vi "Initialize Sim youBot Arm.vi"(8 "error in":errorcluster, 11 "Robot ID":string) -> (0 "error out":errorcluster, 3 "NI_Robotics_KUKA youBot Arm_Sim out":refnum<class "NI_Robotics_KUKA youBot Arm_Sim.lvclass">)   [LabVIEW 2017, in "NI_Robotics_KUKA youBot Host.lvlib" / "NI_Robotics_KUKA youBot Arm_Sim.lvclass"]
uses:
  <vilib>/robotics/KUKA youBot/Basic Device/Arm Sim/NI_Robotics_KUKA youBot Arm_Sim.lvclass
  c:/Program Files (x86)/National Instruments/LabVIEW 2017/vi.lib/robotics/Kinematics/Robot/NI_Robotics_Serial Robot Arm.lvclass
  c:/Program Files (x86)/National Instruments/LabVIEW 2017/vi.lib/robotics/KUKA youBot/Basic Device/Arm/NI_Robotics_KUKA youBot Arm.lvclass
  <vilib>/robotics/Kinematics/DH Dynamic Parameters.ctl
  <vilib>/Analysis/Matrix/Datatypes/RealMatrix.ctl
  <vilib>/robotics/KUKA youBot/Motor/Arm Motor Sim/NI_Robotics_KUKA youBot Arm Motor_Sim.lvclass
  c:/Program Files (x86)/National Instruments/LabVIEW 2017/vi.lib/robotics/KUKA youBot/Motor/Arm Motor/NI_Robotics_KUKA youBot Arm Motor.lvclass
  <vilib>/robotics/KUKA youBot/Basic Device/Gripper Sim/NI_Robotics_KUKA youBot Gripper_Sim.lvclass
  c:/Program Files (x86)/National Instruments/LabVIEW 2017/vi.lib/robotics/KUKA youBot/Basic Device/Gripper/NI_Robotics_KUKA youBot Gripper.lvclass
  <vilib>/Analysis/7linalg.llb/Create Special Real Matrix.vi
  <vilib>/robotics/KUKA youBot/Basic Device/Arm/NI_Robotics_KUKA youBot Arm.lvclass
  <vilib>/robotics/Kinematics/Robot/NI_Robotics_Serial Robot Arm.lvclass
  <vilib>/robotics/Kinematics/NI_Kinematics.lvlib
  <vilib>/Analysis/NI_AALPro.lvlib
  <vilib>/Analysis/Matrix/NI_Matrix.lvlib
  <vilib>/robotics/Kinematics/Link/NI_Robotics_Link.lvclass
panel:
  in  "Arm Index":i32
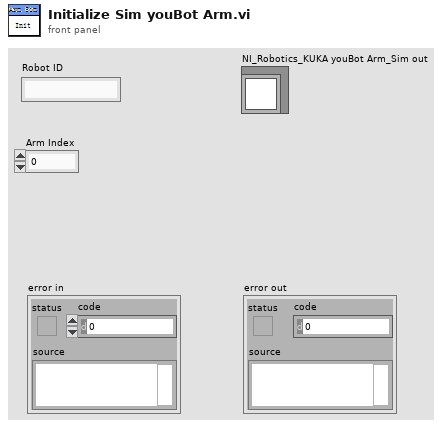
[diagram p1: front panel]
types:
  T1 = typedef "DH Dynamic Parameters.ctl" = cluster{"mass":dbl, "gear ratio":dbl, "motor inertia":dbl, "center of gravity":dbl[], "viscous friction":dbl, "positive coulomb friction":dbl, "negative coulomb friction":dbl, "inertia matrix":T2}
  T2 = typedef "NI_Matrix.lvlib/RealMatrix.ctl" = dbl[][]
  T3 = cluster{"Robot ID":string, "sensor/actuator ID":string}
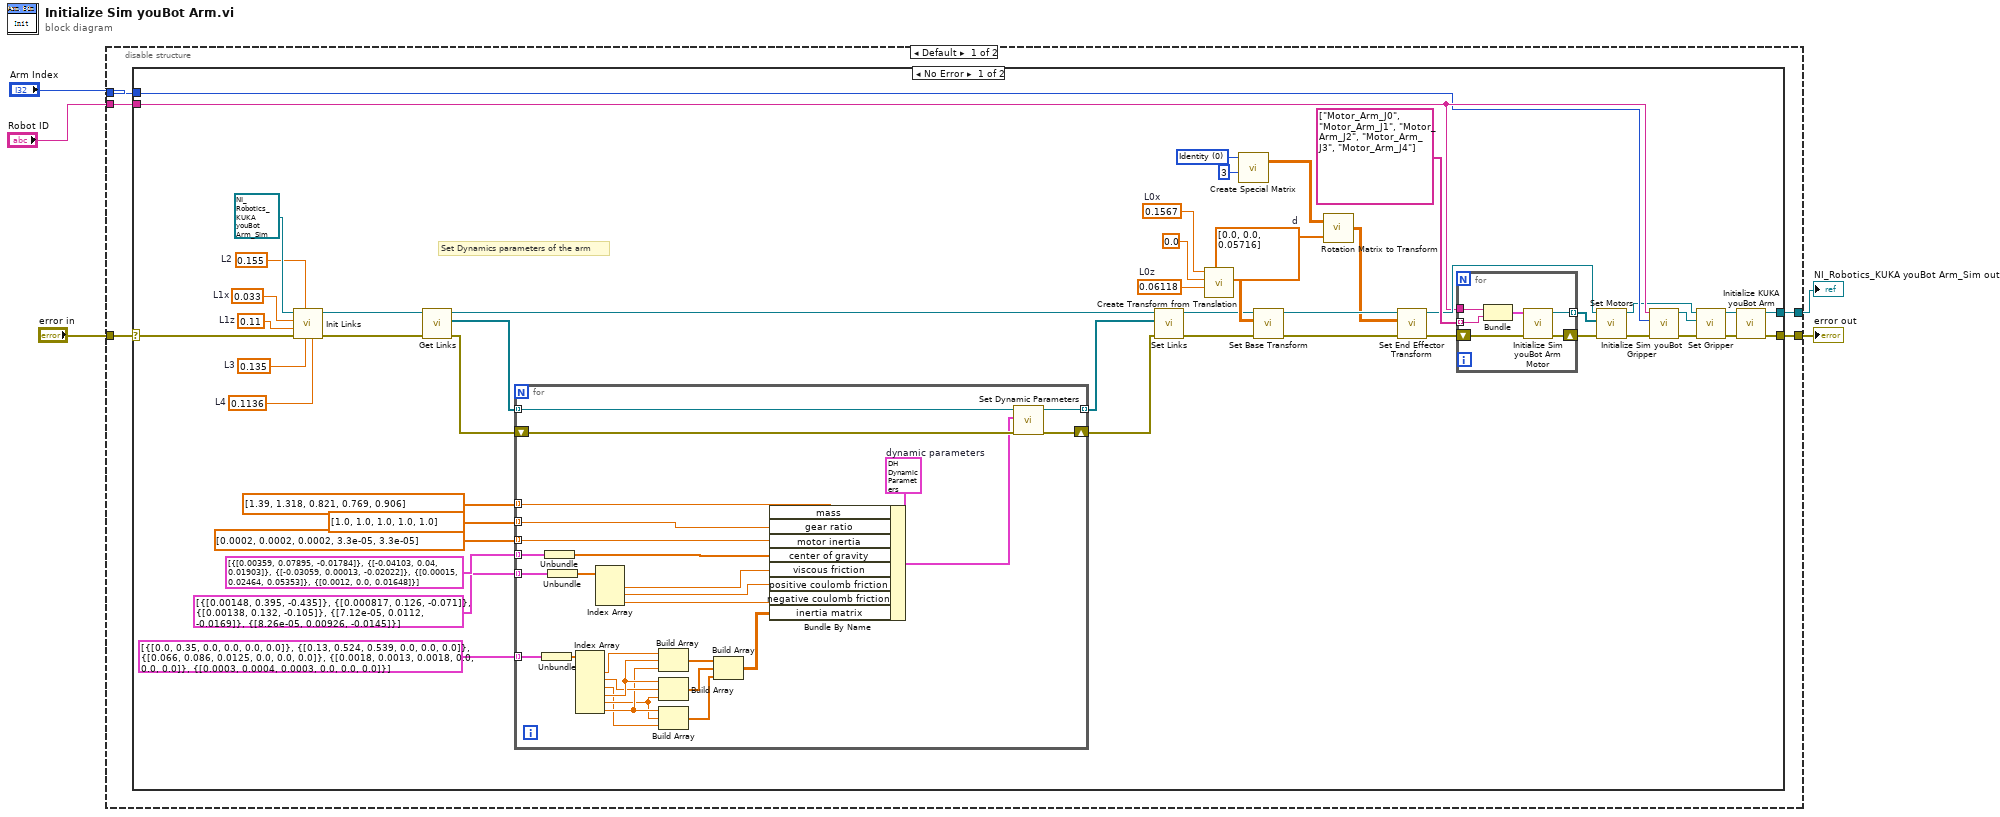
[diagram p0: block diagram]
diagram:
  n1 = disable-structure shown="Default" {
    disable-tunnel: "Robot ID" -> [w10 _]
    disable-tunnel: "error in" -> [w9 _]
    disable-tunnel: [w8 _] -> w3
    disable-tunnel: [w7 _] -> w2
    disable-tunnel: "Arm Index" -> [w6 _]
    frame condition #0 (active) {
      n2 = case shown="No Error" w9 {
        selector: w9 -> [w34 w93]
        tunnel: w10 -> [w42 _]
        tunnel: [w56 w93] -> w8
        tunnel: [w57 _] -> w7
        tunnel: w6 -> [w41 _]
        frame No Error {
          w26 = 0.1136  # L4
          w29 = 0 items=["Identity", "Diagonal", "Toeplitz", "Vandermonde", "Companion", "Hankel", "Hadamard", "Wilkinson", "Hilbert", "Inverse Hilbert", "Rosser", "Pascal"] ("matrix type")
          w44 = dbl[] [0.0, 0.0, 0.05716]  # d
          w30 = 0.135  # L3
          w31 = 0.155  # L2
          w32 = 0.11  # L1z
          w33 = 0.033  # L1x
          w50 = 0.06118  # L0z
          w52 = 0.1567  # L0x
          # "Set Dynamics parameters of the arm"
          n3 = call-dynamic "Init Links.vi"("L4"=w26, "L3"=w30, "L2"=w31, "error in (no error)"=w34, "L1z"=w32, "L1x"=w33, "NI_Robotics_5R Type 1 Serial Arm Class in"=refnum<class "NI_Robotics_KUKA youBot Arm_Sim.lvclass"> refnum ("NI_Robotics_KUKA youBot Host.lvlib:NI_Robotics_KUKA youBot Arm_Sim.lvclass")) -> ("error out"=w18:errorcluster, "NI_Robotics_5R Type 1 Serial Arm Class out"=w19:refnum<class "NI_Robotics_KUKA youBot Arm_Sim.lvclass">)  [unwired: 3 in]
          n4 = call <vilib>:"Get Links.vi"("error in (no error)"=w18, "serial arm in"=w19) -> ("error out"=w17:errorcluster, "links"=w16:refnum<class "NI_Robotics_Link.lvclass">[], "serial arm out"=w11:refnum<class "NI_Robotics_KUKA youBot Arm_Sim.lvclass">)  [unwired: 7 in]
          n5 = for {
            tunnel: w16 -> [w63] mode=indexing
            tunnel: dbl[] [1.39, 1.318, 0.821, 0.769, 0.906] -> [w85] mode=indexing
            tunnel: dbl[] [1.0, 1.0, 1.0, 1.0, 1.0] -> [w84] mode=indexing
            tunnel: dbl[] [0.0002, 0.0002, 0.0002, 3.3e-05, 3.3e-05] -> [w83] mode=indexing
            tunnel: cluster{dbl[]}[] [{[0.00359, 0.07895, -0.01784]}, {[-0.04103, 0.04, 0.01903]}, {[-0.03059, 0.00013, -0.02022]}, {[0.00015, 0.02464, 0.05353]}, {[0.0012, 0.0, 0.01648]}] -> [w82] mode=indexing
            tunnel: cluster{dbl[]}[] [{[0.00148, 0.395, -0.435]}, {[0.000817, 0.126, -0.071]}, {[0.00138, 0.132, -0.105]}, {[7.12e-05, 0.0112, -0.0169]}, {[8.26e-05, 0.00926, -0.0145]}] -> [w80] mode=indexing
            tunnel: cluster{dbl[]}[] [{[0.0, 0.35, 0.0, 0.0, 0.0, 0.0]}, {[0.13, 0.524, 0.539, 0.0, 0.0, 0.0]}, {[0.066, 0.086, 0.0125, 0.0, 0.0, 0.0]}, {[0.0018, 0.0013, 0.0018, 0.0, 0.0, 0.0]}, {[0.0003, 0.0004, 0.0003, 0.0, 0.0, 0.0]}] -> [w66] mode=indexing
            tunnel: [w60] -> w12 mode=indexing
            shift-right: [w59] -> w13
            shift-left: w17 -> [w62]
            w86 = T1 {"mass"=0.0, "gear ratio"=0.0, "motor inertia"=0.0, "center of gravity"=[], "viscous friction"=0.0, "positive coulomb friction"=0.0, "negative coulomb friction"=0.0, "inertia matrix"=[[0.0, 0.0, 0.0], [0.0, 0.0, 0.0], [0.0, 0.0, 0.0]]}  # dynamic parameters
            n6 = Unbundle(w66) -> (w65:dbl[])
            n7 = Unbundle(w82) -> (w81:dbl[])
            n8 = Unbundle(w80) -> (w79:dbl[])
            n9 = Index Array(array=w65) -> (element #1=w75:dbl, element #2=w73:dbl, element #3=w70:dbl, element #4=w74:dbl, element #5=w71:dbl, element #6=w72:dbl)  [unwired: 6 in]
            n10 = Index Array(array=w79) -> (element #1=w78:dbl, element #2=w77:dbl, element #3=w76:dbl)  [unwired: 3 in]
            n11 = Build Array(w75, w74, w72) -> (w69:dbl[])
            n12 = Build Array(w74, w73, w71) -> (w68:dbl[])
            n13 = Build Array(w72, w71, w70) -> (w67:dbl[])
            n14 = Build Array(w69, w68, w67) -> (w64:dbl[][])
            n15 = Bundle By Name(cluster=w86, "mass"=w85, "gear ratio"=w84, "motor inertia"=w83, "center of gravity"=w81, "viscous friction"=w78, "positive coulomb friction"=w77, "negative coulomb friction"=w76, "inertia matrix"=w64) -> (w61:T1)
            n16 = call <vilib>:"Set Dynamic Parameters.vi"("error in (no error)"=w62, "dynamic parameters"=w61, "link in"=w63) -> ("error out"=w59:errorcluster, "link out"=w60:refnum<class "NI_Robotics_Link.lvclass">)  [unwired: 7 in]
          }
          n17 = call <vilib>:"Set Links.vi"("error in (no error)"=w13, "links"=w12, "serial arm in"=w11) -> ("error out"=w14:errorcluster, "serial arm out"=w15:refnum<class "NI_Robotics_KUKA youBot Arm_Sim.lvclass">)  [unwired: 7 out]
          n18 = call <vilib>:"Create Transform from Translation.vi"("z"=w50, "y"=0.0, "x"=w52) -> ("transform"=w53:T2)  [unwired: 8 in]
          n19 = call-poly <vilib>:"Create Special Matrix.vi"("matrix type"=w29, "matrix size"=3) -> ("Special Matrix"=w27:T2)  [unwired: 3 in, 1 out]
          n20 = call <vilib>:"Set Base Transform.vi"("error in (no error)"=w14, "base transform"=w53, "serial arm in"=w15) -> ("error out"=w49:errorcluster, "serial arm out"=w47:refnum<class "NI_Robotics_KUKA youBot Arm_Sim.lvclass">)  [unwired: 7 in]
          n21 = call <vilib>:"Rotation Matrix to Transform.vi"("translation vector"=w44, "rotation matrix"=w27) -> ("transform"=w45:T2)
          n22 = call <vilib>:"Set End Effector Transform.vi"("error in (no error)"=w49, "end effector transform"=w45, "serial arm in"=w47) -> ("error out"=w48:errorcluster, "serial arm out"=w46:refnum<class "NI_Robotics_KUKA youBot Arm_Sim.lvclass">)  [unwired: 7 in]
          n23 = for {
            tunnel: string[] ["Motor_Arm_J0", "Motor_Arm_J1", "Motor_Arm_J2", "Motor_Arm_J3", "Motor_Arm_J4"] -> [w91] mode=indexing
            tunnel: w42 -> [w92]
            shift-right: [w88] -> w54
            shift-left: w48 -> [w89]
            tunnel: [w87] -> w58 mode=indexing
            n24 = Bundle("Robot ID"=w92, "sensor/actuator ID"=w91) -> (w90:T3)  [unwired: 1 in]
            n25 = call <vilib>:"Initialize Sim youBot Arm Motor.vi"("error in (no error)"=w89, "device ID"=w90) -> ("error out"=w88:errorcluster, "simulated KUKA youBot arm motor out"=w87:refnum<class "NI_Robotics_KUKA youBot Arm Motor_Sim.lvclass">)  [unwired: 8 in]
          }
          n26 = call <vilib>:"Set Motors.vi"("error in (no error)"=w54, "motors"=w58, "KUKA youBot arm in"=w46) -> ("error out"=w43:errorcluster, "KUKA youBot arm out"=w38:refnum<class "NI_Robotics_KUKA youBot Arm_Sim.lvclass">)  [unwired: 7 in]
          n27 = call <vilib>:"Initialize Sim youBot Gripper.vi"("error in (no error)"=w43, "arm index"=w41, "robot ID"=w42) -> ("error out"=w40:errorcluster, "simulated KUKA youBot gripper out"=w39:refnum<class "NI_Robotics_KUKA youBot Gripper_Sim.lvclass">)  [unwired: 7 in]
          n28 = call-dynamic "Set Gripper.vi"("error in (no error)"=w40, "KUKA youBot gripper"=w39, "KUKA youBot arm in"=w38) -> ("error out"=w36:errorcluster, "KUKA youBot arm out"=w37:refnum<class "NI_Robotics_KUKA youBot Arm_Sim.lvclass">)  [unwired: 7 in]
          n29 = call <vilib>:"Initialize KUKA youBot Arm.vi"("error in (no error)"=w36, "KUKA youBot arm in"=w37) -> ("error out"=w56:errorcluster, "KUKA youBot arm out"=w57:refnum<class "NI_Robotics_KUKA youBot Arm_Sim.lvclass">)  [unwired: 8 in]
        }
        frame Error {
        }
      }
    }
    frame condition #1 {
    }
  }
  "error out" <- w3
  "NI_Robotics_KUKA youBot Arm_Sim out" <- w2
